vi "6-AlarmStatus.vi"(8 "error in (no error)":errorcluster caption="错误输入（无错误）", 9 "AlarmValue":bool, 10 "AlarmIndex":T1, 11 "Step":enum16{"Initial", "Write", "Read"}(ring)) -> (0 "error out":errorcluster caption="错误输出", 2 "AlarmValue Out":bool[](array[boolean]))   [LabVIEW 2017]
uses:
  Ctrls/AlarmIndex.ctl
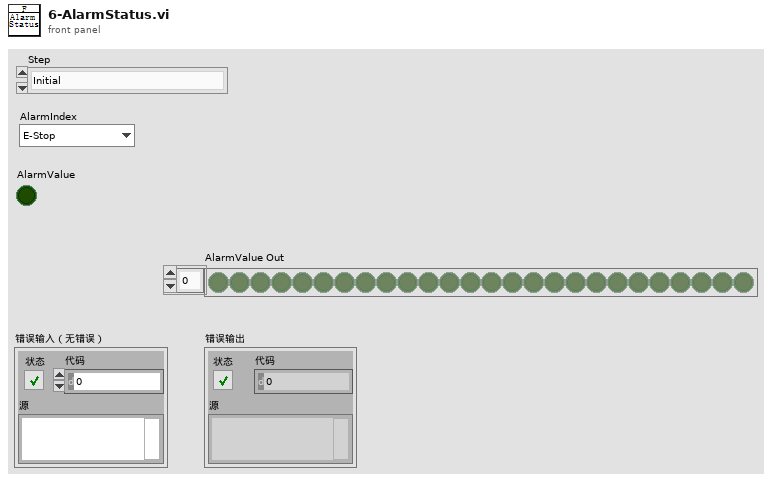
[diagram p1: front panel]
types:
  T1 = typedef "AlarmIndex.ctl" = enum16{"E-Stop", "Safety light grid", "UUT Sealing Cylinder HomePoint", "UUT Sealing Cylinder WorkPoint", "Orifice fixed Cylinder L HomePoint", "Orifice fixed Cylinder L WorkPoint", "Orifice fixed Cylinder R HomePoint", "Orifice fixed Cylinder R WorkPoint", "UUT Cylinder HomePoint", "UUT Cylinder WorkPoint", "Carrier fixed Cylinder L HomePoint", "Carrier fixed Cylinder L WorkPoint", "Carrier fixed Cylinder R HomePoint", "Carrier fixed Cylinder R WorkPoint", "Probe Cylinder HomePoint", "Probe Cylinder WorkPoint", "Motor Error", "Test Error"}
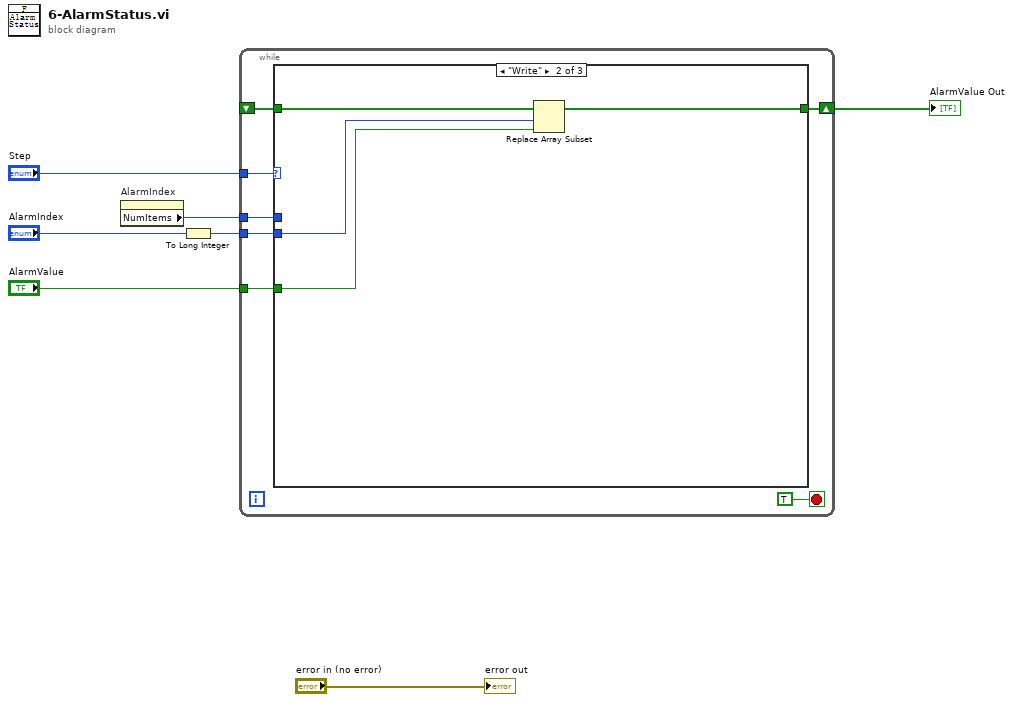
[diagram p0: block diagram]
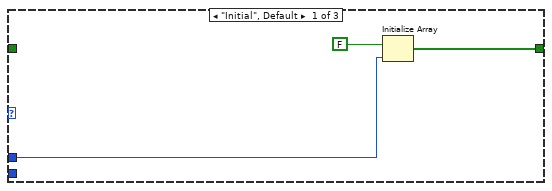
[diagram p2: hidden frame]
diagram:
  n1 = property on="AlarmIndex" class="Enum (strict)"() -> ("NumItems"=w1:u32)  [unwired: 2 in, 2 out]
  n2 = To Long Integer(number="AlarmIndex") -> (32bit integer=w3:i32)
  n3 = while {
    tunnel: "Step" -> [w13]
    shift-right: [w12] -> w2
    shift-left: _ -> [w11]
    tunnel: w3 -> [w10]
    tunnel: "AlarmValue" -> [w9]
    tunnel: w1 -> [w8]
    stop <- TRUE stop-if-true
    n4 = case shown="\"Write\"" w13 {
      tunnel: [w16 w20 w22] -> w12
      tunnel: w11 -> [_ w21 w22]
      tunnel: w10 -> [_ w19 _]
      tunnel: w9 -> [_ w18 _]
      tunnel: w8 -> [w15 _ _]
      frame "Initial", Default {
        n5 = Initialize Array(FALSE, w15) -> (w16:bool[])
      }
      frame "Write" {
        n6 = Replace Array Subset ("替换数组子集")(array=w21, new element=w18, index=w19) -> (w20:bool[])
      }
      frame "Read" {
      }
    }
  }
  "AlarmValue Out" <- w2
  "error out" <- "error in (no error)"
